vi "DashboardGetPolyscopeVersion.vi"(8 "Dashboard":refnum<k24>, 11 "error in":errorcluster) -> (0 "Response":cluster{"Message":string, "Succeed":bool}, 1 "Version":T1, 3 "error out":errorcluster)   [LabVIEW 2011, in "UnderAutomation.UniversalRobots.lvlib"]
uses:
  UnderAutomation.UniversalRobots.lvlib
  C:/Users/fg/Documents/UniversalRobots.vi/LabVIEW_2024/UnderAutomation.UniversalRobots/lib/UnderAutomation.UniversalRobots.dll
  LabVIEW_2024/UnderAutomation.UniversalRobots/lib/UnderAutomation.UniversalRobots.dll
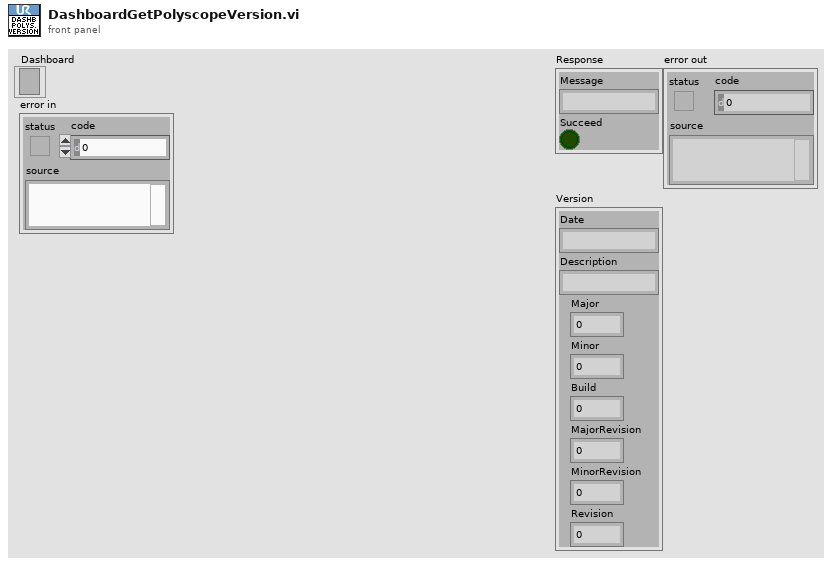
[diagram p1: front panel]
types:
  T1 = cluster{"Date":string, "Description":string, "Major":i32, "Minor":i32, "Build":i32, "MajorRevision":i16, "MinorRevision":i16, "Revision":i32}
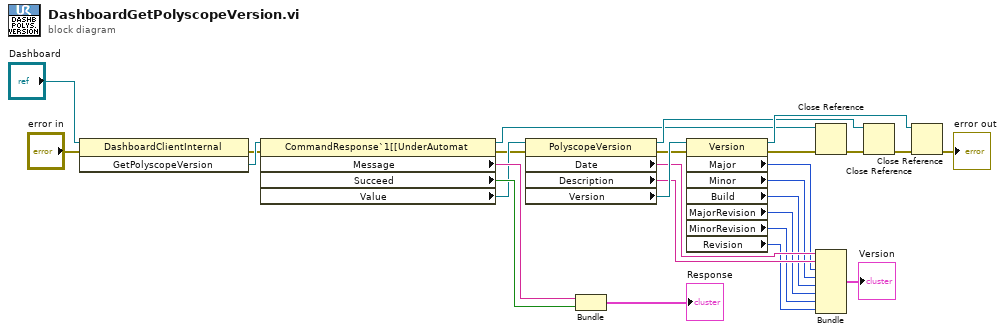
[diagram p0: block diagram]
diagram:
  n1 = invoke class="DashboardClientInternal" method="GetPolyscopeVersion"(reference="Dashboard", error in="error in") -> (error out=w21:errorcluster, "GetPolyscopeVersion"=w26:refnum<k24>)  [unwired: 1 in, 1 out]
  n2 = property class="CommandResponse`1[[UnderAutomat"(reference=w26, error in=w21) -> (reference out=w1:refnum<k24>, error out=w9:errorcluster, "Message"=w25:string, "Succeed"=w24:bool, "Value"=w20:refnum<k24>)
  n3 = property class="PolyscopeVersion"(reference=w20, error in=w9) -> (reference out=w2:refnum<k24>, error out=w8:errorcluster, "Date"=w18:string, "Description"=w17:string, "Version"=w19:refnum<k24>)
  n4 = Bundle("Message"=w25, "Succeed"=w24) -> (→"Response":cluster{"Message":string, "Succeed":bool})  [unwired: 1 in]
  n5 = property class="Version"(reference=w19, error in=w8) -> (reference out=w3:refnum<k24>, error out=w7:errorcluster, "Major"=w16:i32, "Minor"=w15:i32, "Build"=w14:i32, "MajorRevision"=w13:i16, "MinorRevision"=w12:i16, "Revision"=w11:i32)
  n6 = Close Reference(reference=w1, error in (no error)=w7) -> (error out=w6:errorcluster)
  n7 = Bundle("Date"=w18, "Description"=w17, "Major"=w16, "Minor"=w15, "Build"=w14, "MajorRevision"=w13, "MinorRevision"=w12, "Revision"=w11) -> (→"Version":T1)  [unwired: 1 in]
  n8 = Close Reference(reference=w2, error in (no error)=w6) -> (error out=w5:errorcluster)
  n9 = Close Reference(reference=w3, error in (no error)=w5) -> (error out=→"error out":errorcluster)
